vi "FdxCmdTxEDEWriteCvi.vi"(8 "error in":errorcluster, 9 "Input Cluster":T1, 10 "EDEHandle":u32, 11 "InstrumentHandle":u32) -> (0 "error out":errorcluster, 1 "BytesWritten":u32, 3 "InstrumentHandle":u32)   [LabVIEW 2020, in "AIM664LV.lvlib"]
doc: "This function is used to write a pure message to an EDE port. This port can be a sampling or a queuing port. If the data size is not applicable for the data size associated to this port, this function will return an error.\nThis function can be used to inject EDE errors into the written message. \nFor sampling ports this function initializes / modifies data contents. \nFor queuing ports a transmission is initiated when data is written to a UDP port. \nThis function can be used if the transmitter is running or not running. \nFor sampling ports this function should be called before the port is started to initialize the data contents of the sampling port."
uses:
  AIM664LV.lvlib
  AFDX_LibraryAdmin/FdxGlobalDllPath.vi
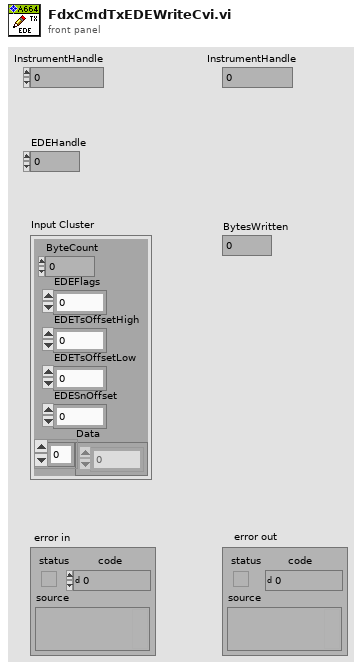
[diagram p1: front panel]
types:
  T1 = cluster{"ByteCount":u32, "Data":dbl[], "EDEFlags":u32, "EDETsOffsetHigh":u32, "EDETsOffsetLow":u32, "EDESnOffset":u16}
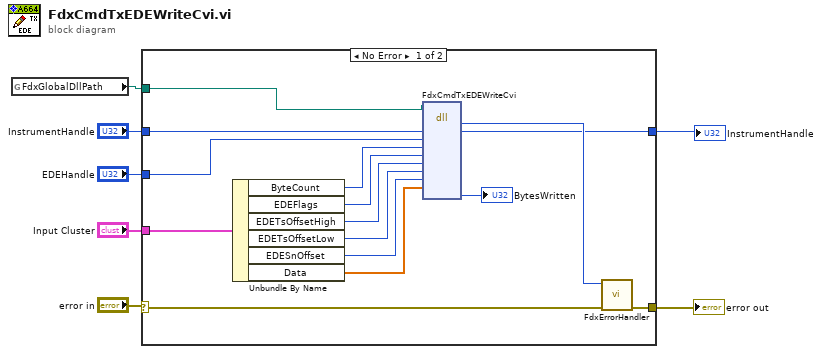
[diagram p0: block diagram]
diagram:
  n1 = global read "FdxGlobalDllPath.vi" "FdxGlobalDllPath"() -> (w5:path)
  n2 = case shown="No Error" "error in" {
    selector: "error in" -> [w21 w24]
    tunnel: [w22 w24] -> w7
    tunnel: w5 -> [w12 _]
    tunnel: "InstrumentHandle" -> [w11 w23]
    tunnel: [w10 w23] -> w3
    tunnel: "Input Cluster" -> [w9 _]
    tunnel: "EDEHandle" -> [w8 _]
    frame No Error {
      n3 = Unbundle By Name(w9) -> ("ByteCount"=w19:u32, "EDEFlags"=w18:u32, "EDETsOffsetHigh"=w16:u32, "EDETsOffsetLow"=w15:u32, "EDESnOffset"=w14:u16, "Data"=w13:dbl[])
      n4 = dll-call lib="aim_fdx.19.dll" fn="FdxCmdTxEDEWriteCvi"(path in=w12, "InstrumentHandle"=w11, "EDEHandle"=w8, "ByteCount"=w19, "EDEFlags"=w18, "EDETsOffsetHigh"=w16, "EDETsOffsetLow"=w15, "EDESnOffset"=w14, "Data"=w13) -> ("status"=w20:i32, "InstrumentHandle"=w10:u32, "BytesWritten"=→"BytesWritten":u32)  [unwired: 7 in, 5 out]
      n5 = call "FdxErrorHandler.vi"("error in"=w21, "AIM Error"=w20) -> ("error out"=w22:errorcluster)  [unwired: 9 in]
    }
    frame Error {
    }
  }
  "error out" <- w7
  "InstrumentHandle" <- w3
